vi "CSV to HTTP.vi"(1 "Delimiter":string=",") -> (0 "HTML Table":string)   [LabVIEW 2019, in "Useful HTTP VIs.lvlib"]
uses:
  Useful HTTP VIs.lvlib
  <vilib>/Utility/file.llb/Read Delimited Spreadsheet (string).vi
  <vilib>/JDP Science/JSONtext/Variant to JSON Text.vi
  <vilib>/JDP Science/JSONtext/LVClass Serializer/JSONtext LVClass Serializer.lvclass
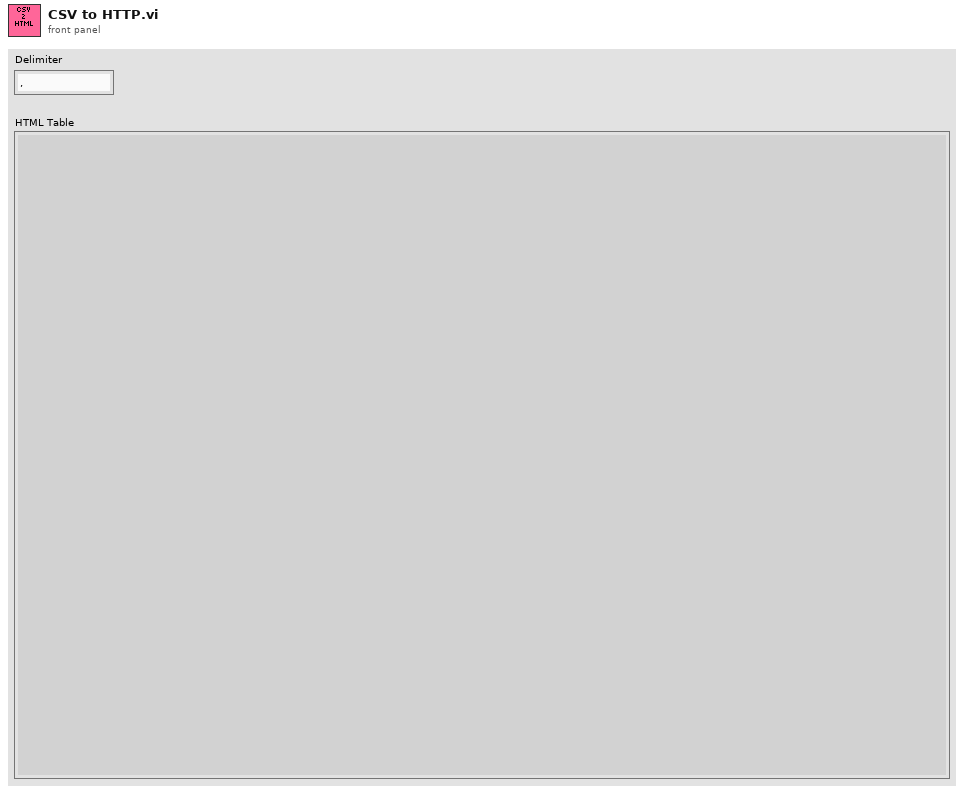
[diagram p1: front panel]
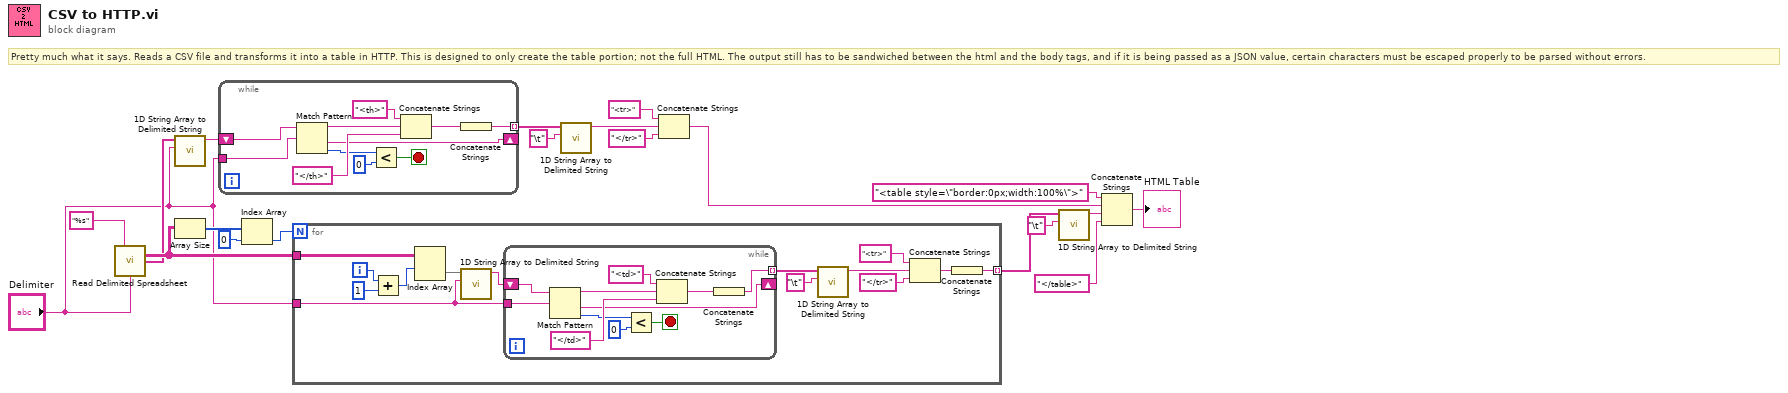
[diagram p0: block diagram]
diagram:
  # "Pretty much what it says. Reads a CSV file and transforms it into a table in HTTP. This is designed to only create the table portion; not the full HTML. The output still has to be sandwiched between the html and the body tags, and if it is being passed as a JSON value, certain characters must be escaped properly to be parsed without errors."
  n1 = call-poly <vilib>:"Read Delimited Spreadsheet.vi"("format (%s)"="%s", "delimiter (\\t)"="Delimiter") -> ("all rows"=w15:string[][], "first row"=w10:string[])  [unwired: 8 in, 4 out]
  n2 = call <vilib>:"1D String Array to Delimited String.vi"("delimiter"="Delimiter", "string array"=w10) -> ("delimited string"=w9:string)  [unwired: 9 in]
  n3 = Array Size(array=w15) -> (size(s)=w17:i32[])
  n4 = while {
    tunnel: [w24] -> w4 mode=indexing
    shift-right: [w23] -> _
    shift-left: w9 -> [w22]
    tunnel: "Delimiter" -> [w21]
    stop <- w26 stop-if-true
    n5 = Match Pattern(string=w22, regular expression=w21) -> (before substring=w31:string, after substring=w23:string, offset past match=w28:i32)  [unwired: 1 in, 1 out]
    n6 = Less?(x=w28, y=0) -> (x < y?=w26:bool)
    n7 = Concatenate Strings("<th>" ("string"), w31, "</th>" ("string")) -> (w25:string)
    n8 = Concatenate Strings(w25) -> (w24:string)
  }
  n9 = Index Array(array=w17, index=0) -> (element=w11:i32)
  n10 = for {
    N: w11 -> [_]
    tunnel: "Delimiter" -> [w45]
    tunnel: [w37] -> w19 mode=indexing
    tunnel: w15 -> [w36]
    i -> [w33]
    n11 = Add(x=w33, y=1) -> (x+y=w32:i32)
    n12 = Index Array(array=w36, index (row)=w32) -> (element=w35:string[])  [unwired: 1 in]
    n13 = call <vilib>:"1D String Array to Delimited String.vi"("delimiter"=w45, "string array"=w35) -> ("delimited string"=w44:string)  [unwired: 9 in]
    n14 = while {
      shift-right: [w51] -> _
      shift-left: w44 -> [w56]
      tunnel: w45 -> [w52]
      tunnel: [w46] -> w43 mode=indexing
      stop <- w48 stop-if-true
      n15 = Match Pattern(string=w56, regular expression=w52) -> (before substring=w55:string, after substring=w51:string, offset past match=w50:i32)  [unwired: 1 in, 1 out]
      n16 = Less?(x=w50, y=0) -> (x < y?=w48:bool)
      n17 = Concatenate Strings("<td>" ("string"), w55, "</td>" ("string")) -> (w47:string)
      n18 = Concatenate Strings(w47) -> (w46:string)
    }
    n19 = call <vilib>:"1D String Array to Delimited String.vi"("delimiter"="\t", "string array"=w43) -> ("delimited string"=w40:string)  [unwired: 9 in]
    n20 = Concatenate Strings("<tr>" ("string"), w40, "</tr>" ("string")) -> (w38:string)
    n21 = Concatenate Strings(w38) -> (w37:string)
  }
  n22 = call <vilib>:"1D String Array to Delimited String.vi"("delimiter"="\t", "string array"=w4) -> ("delimited string"=w6:string)  [unwired: 9 in]
  n23 = Concatenate Strings("<tr>" ("string"), w6, "</tr>" ("string")) -> (w3:string)
  n24 = call <vilib>:"1D String Array to Delimited String.vi"("delimiter"="\t", "string array"=w19) -> ("delimited string"=w12:string)  [unwired: 9 in]
  n25 = Concatenate Strings("<table style=\"border:0px;width:100%\">" ("string"), w3, w12, "</table>" ("string")) -> (→"HTML Table":string)
